vi "Mute.vi"(7 "Direction":T1, 8 "error in (no error)":errorcluster, 9 "Mute? (T)":bool=TRUE, 10 "Index":i32, 11 "VoiceMeeterRemote in":refnum<class "VoiceMeeterRemote.lvclass">) -> (0 "error out":errorcluster, 3 "VoiceMeeterRemote out":refnum<class "VoiceMeeterRemote.lvclass">)   [LabVIEW 2020, in "VoiceMeeterRemote.lvlib" / "VoiceMeeterRemote.lvclass"]
doc: "Sets the mute state of the specified input or output index."
uses:
  VoiceMeeterRemote.lvclass
  Direction.ctl
  VoiceMeeterRemote.lvlib
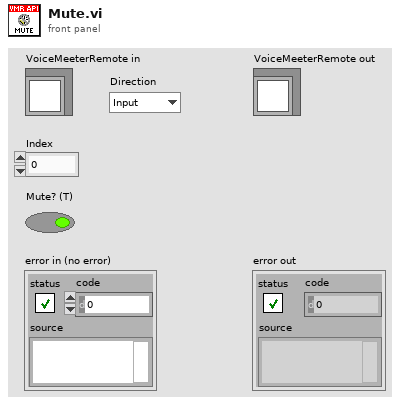
[diagram p1: front panel]
types:
  T1 = typedef "VoiceMeeterRemote.lvlib/Direction.ctl" = enum16{"Input", "Output"}
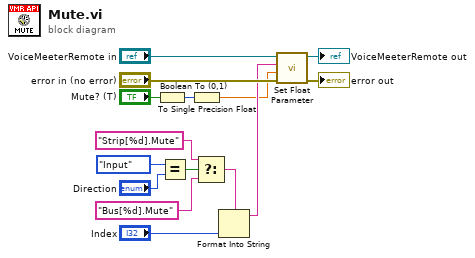
[diagram p0: block diagram]
diagram:
  n1 = Boolean To (0,1)(Boolean="Mute? (T)") -> (0, 1=w2:i16)
  n2 = Equal?(x=Direction."Input", y="Direction") -> (x = y?=w12:bool)
  n3 = To Single Precision Float(number=w2) -> (single precision float=w1:sgl)
  n4 = Select(t="Strip[%d].Mute", s=w12, f="Bus[%d].Mute") -> (s? t:f=w9:string)
  n5 = Format Into String(format string=w9, "Index") -> (resulting string=w6:string)  [unwired: 2 in, 1 out]
  n6 = call "Set Float Parameter.vi"("error in (no error)"="error in (no error)", "Value"=w1, "Parameter Name"=w6, "VoiceMeeterRemote in"="VoiceMeeterRemote in") -> ("error out"=→"error out":errorcluster, "VoiceMeeterRemote out"=→"VoiceMeeterRemote out":refnum<class "VoiceMeeterRemote.lvclass">)  [unwired: 6 in]
